vi "test.vi"() -> ()   [LabVIEW 2011]
panel:
  out "Real 2":dbl
  out "Real":dbl
  out "Intensity Graph":dbl[][](graph)
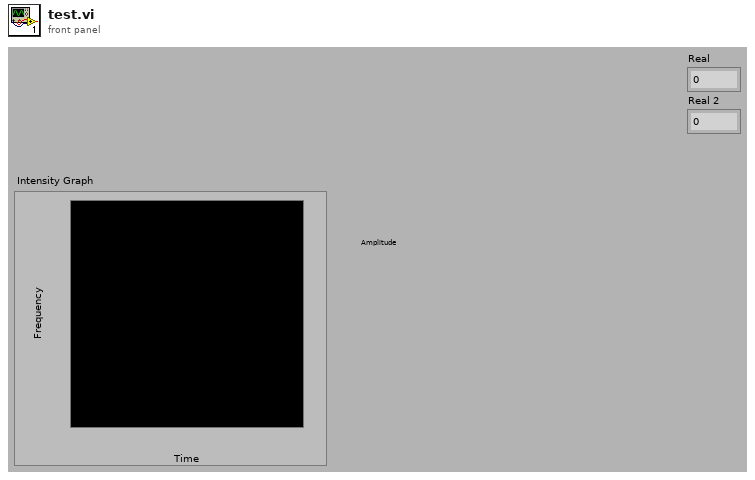
[diagram p1: front panel]
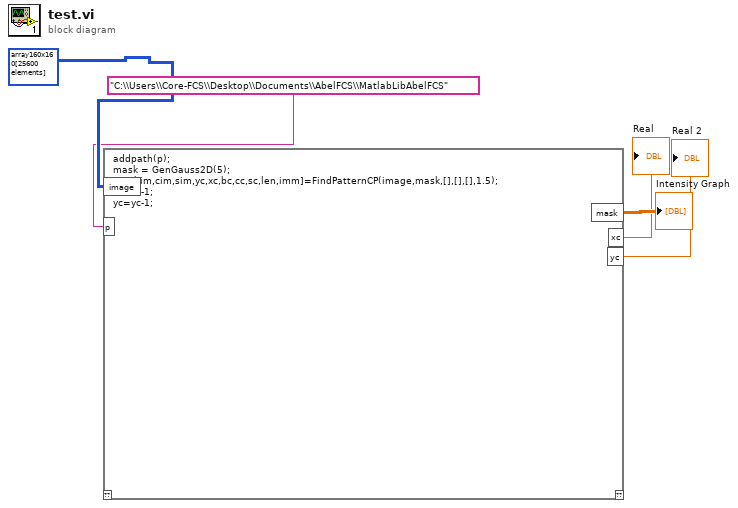
[diagram p0: block diagram]
diagram:
  n1 = script code="addpath(p);\nmask = GenGauss2D(5);\n[err,bim,cim,sim,yc,xc,bc,cc,sc,len,imm]=FindPatternCP(image,mask,[],[],[],1.5);\nxc=xc-1;\nyc=yc-1;"("image"=i32[][] array160x160[25600 elements] ("Image"), "p"="C:\\Users\\Core-FCS\\Desktop\\Documents\\AbelFCS\\MatlabLibAbelFCS" ("String")) -> ("mask"=→"Intensity Graph":dbl[][], "xc"=→"Real":dbl, "yc"=→"Real 2":dbl)  [unwired: 1 in, 1 out]
